vi "UDP3rtglob.vi"() -> ()   [LabVIEW 2009]
uses:
  UDP 3.ctl
panel:
  in  "UDP 3":T1
  in  "stop":bool
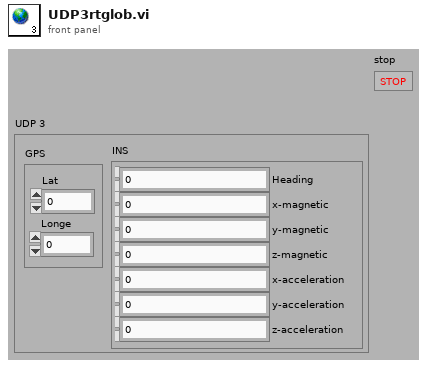
[diagram p1: front panel]
types:
  T1 = typedef "UDP 3.ctl" = cluster{"GPS":cluster{"Lat":dbl, "Longe":dbl}, "INS":cluster{"Heading":dbl, "x-magnetic":dbl, "y-magnetic":dbl, "z-magnetic":dbl, "x-acceleration":dbl, "y-acceleration":dbl, "z-acceleration":dbl}}
diagram:
